vi "Configure Route Multiple.vi"(0 "VISA resource name":refnum<visa-resource-name>, 1 "Operation (0: Open All)":u16(ring) items=["Open All", "Open", "Close"], 2 "Channels (Empty)":i32[](array[numeric]), 5 "error in (no error)":errorcluster) -> (14 "VISA resource name out":refnum<visa-resource-name>, 19 "error out":errorcluster)   [LabVIEW 2013, in "Keithley 2000.lvlib"]
doc: "This VI controls the switch functionality of an internal or external scanner card. It can be used to open or close one or more channels.\n\nNote:\nThis is a polymorphic VI. You can wire a single channel number or an array of channel numbers to configure multiple channels at once."
uses:
  Keithley 2000.lvlib
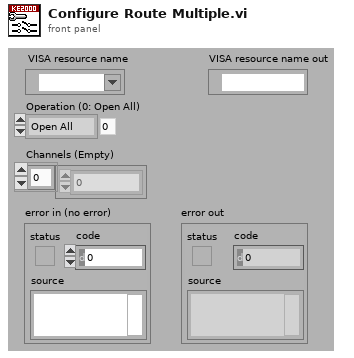
[diagram p1: front panel]
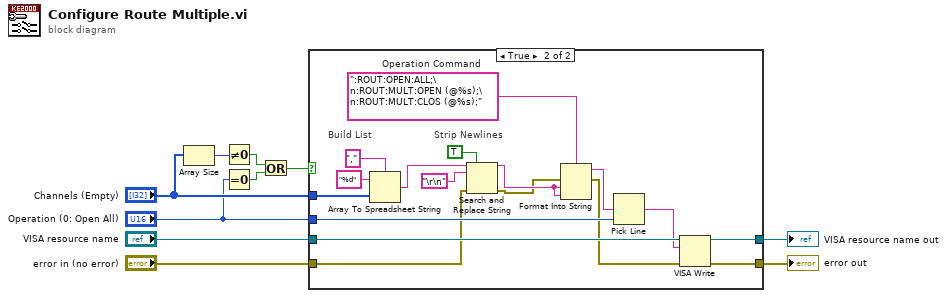
[diagram p0: block diagram]
diagram:
  n1 = Array Size(array="Channels (Empty)") -> (size(s)=w5:i32)
  n2 = Not Equal To 0?(x=w5) -> (x != 0?=w3:bool)
  n3 = Equal To 0?(x="Operation (0: Open All)") -> (x = 0?=w2:bool)
  n4 = Or(x=w3, y=w2) -> (x .or. y?=w1:bool)
  n5 = case shown="True" w1 {
    tunnel: "VISA resource name" -> [w12 w29]
    tunnel: "error in (no error)" -> [w11 w15]
    tunnel: [w12 w28] -> w8
    tunnel: [w11 w27] -> w7
    tunnel: "Operation (0: Open All)" -> [_ w24]
    tunnel: "Channels (Empty)" -> [_ w20]
    frame False {
    }
    frame True {
      w26 = ":ROUT:OPEN:ALL;\n:ROUT:MULT:OPEN (@%s);\n:ROUT:MULT:CLOS (@%s);"  # Operation Command
      # "Strip Newlines"
      # "Build List"
      n6 = Array To Spreadsheet String(delimiter (Tab)=",", array=w20, 3:"%d" ("format string")) -> (spreadsheet string=w18:string)
      n7 = Search and Replace String(replace all?=TRUE ("replace all? (F)"), input string=w18, search string="\r\n", error in=w15) -> (result string=w17:string, error out=w14:errorcluster)  [unwired: 4 in, 2 out]
      n8 = Format Into String(format string=w26, error in=w14, w17, w17) -> (resulting string=w25:string, error out=w13:errorcluster)  [unwired: 1 in]
      n9 = Pick Line(multi-line string=w25, line index=w24) -> (output string=w23:string)  [unwired: 1 in]
      n10 = VISA Write(VISA resource name=w29, write buffer=w23, error in (no error)=w13) -> (VISA resource name out=w28:refnum<visa-resource-name>, error out=w27:errorcluster)  [unwired: 1 out]
    }
  }
  "error out" <- w7
  "VISA resource name out" <- w8
